vi "CAN Uninitialize.vi"(8 "error in (no error)":errorcluster caption="错误输入（无错误）", 11 "Channel":u8) -> (0 "error out":errorcluster caption="错误输出", 3 "function return":u32)   [LabVIEW 2021]
doc: "TPCANStatus __stdcall CAN_Uninitialize(\n TPCANHandle Channel);"
uses:
  PCANBasic.dll
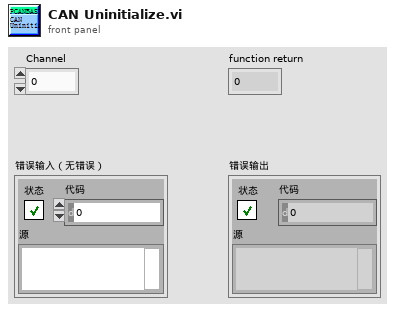
[diagram p1: front panel]
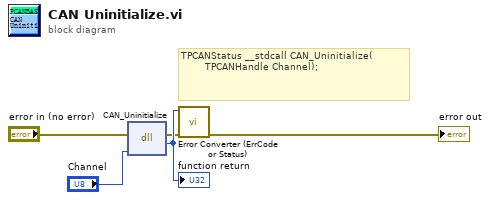
[diagram p0: block diagram]
diagram:
  # "TPCANStatus __stdcall CAN_Uninitialize(\n        TPCANHandle Channel);"
  n1 = dll-call lib="D:/ON LINE WORK/LabVIEW/PCAN/PCAN 1.6(2021)/PCANBasic.*" fn="CAN_Uninitialize"(error in="error in (no error)", "Channel"="Channel") -> (error out=w2:errorcluster, "返回类型"=w5:u32)  [unwired: 3 in, 1 out]
  "function return" <- w5
  n2 = call "Error Converter (ErrCode or Status).vi"("error in (no error)"=w2, "error code"=w5) -> ("error out"=→"error out":errorcluster)  [unwired: 9 in]
